vi "Diff_Drive_Sim.vi"() -> ()   [LabVIEW 2019]
uses:
  Sim_Diff_Drive_Globals.vi
panel:
  out "IMU angle(Degrees)":dbl
  out "Left Wheel Position":dbl
  out "Right Wheel Position":dbl
  in  "turning_friction":dbl
  in  "J":dbl
  in  "initial IMU value(degrees)":dbl=0.01
  in  "wheel_base_length":dbl=0.01
  in  "wheel_mass":dbl
  in  "Wheel_friction":dbl
  in  "kinematics delta t (s)":dbl=0.01
  in  "left_wheel_init":dbl
  in  "right_wheel_init":dbl
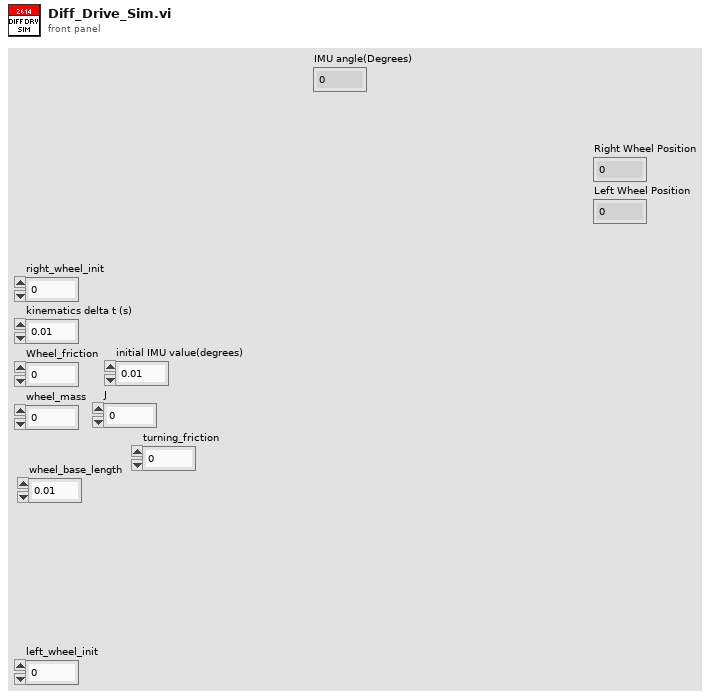
[diagram p1: front panel]
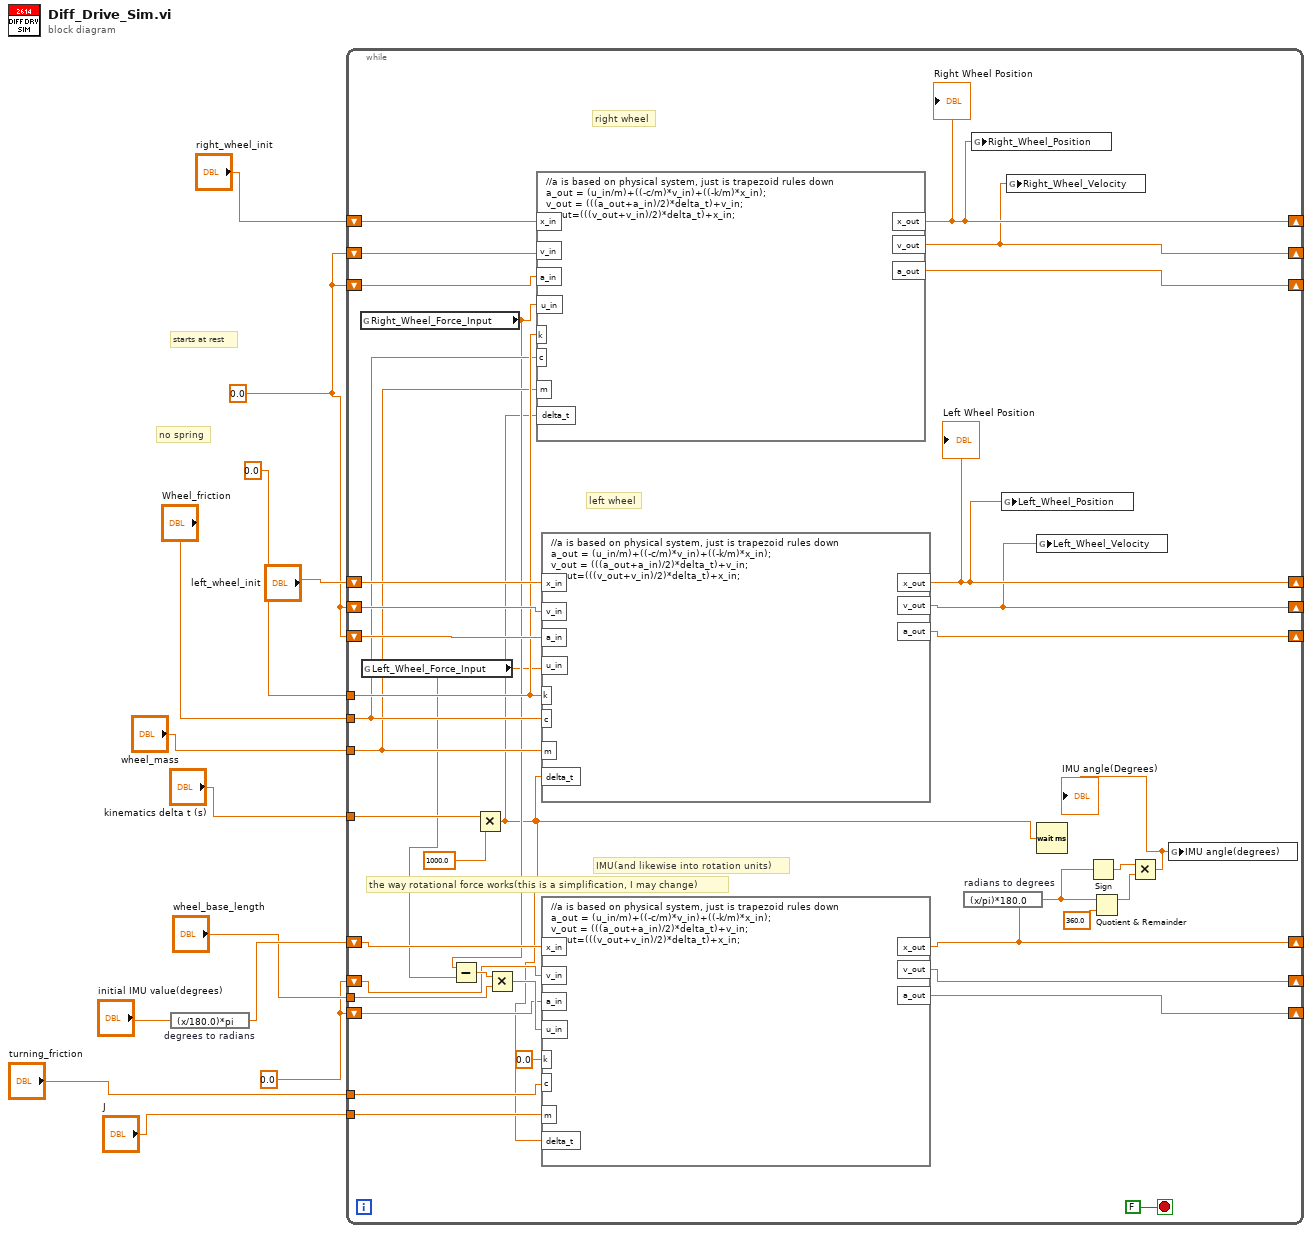
[diagram p0: block diagram]
diagram:
  w3 = 0.0 ("initial IMU value(degrees)")
  w11 = 0.0 ("input variable")
  # "no spring"
  # "starts at rest"
  n1 = expression code="(x/180.0)*pi" "degrees to radians"("initial IMU value(degrees)") -> (w5:dbl)
  n2 = while {
    shift-right: [w37] -> _
    shift-left: w11 -> [w49]
    shift-right: [w35] -> _
    shift-left: w11 -> [w48]
    shift-right: [w44] -> _
    shift-left: w11 -> [w47]
    shift-right: [w45] -> _
    shift-left: w11 -> [w46]
    shift-right: [w38] -> _
    shift-left: "right_wheel_init" -> [w51]
    shift-right: [w36] -> _
    shift-left: "left_wheel_init" -> [w50]
    tunnel: 0.0 ("input variable") -> [w43]
    tunnel: "kinematics delta t (s)" -> [w41]
    tunnel: "Wheel_friction" -> [w40]
    tunnel: "wheel_mass" -> [w39]
    shift-right: [w19] -> _
    shift-left: w5 -> [w34]
    shift-right: [w26] -> _
    shift-left: w3 -> [w28]
    shift-right: [w25] -> _
    shift-left: w3 -> [w27]
    tunnel: "wheel_base_length" -> [w30]
    tunnel: "J" -> [w24]
    tunnel: "turning_friction" -> [w22]
    stop <- FALSE stop-if-true
    # "the way rotational force works(this is a simplification, I may change)"
    # "IMU(and likewise into rotation units)"
    # "left wheel"
    # "right wheel"
    n3 = global read "Sim_Diff_Drive_Globals.vi" "Right_Wheel_Force_Input"() -> (w33:dbl)
    n4 = global read "Sim_Diff_Drive_Globals.vi" "Left_Wheel_Force_Input"() -> (w32:dbl)
    n5 = Subtract(x=w33, y=w32) -> (x-y=w31:dbl)
    n6 = Multiply(x=w41, y=1000.0) -> (x*y=w21:dbl)
    n7 = Multiply(x=w31, y=w30) -> (x*y=w29:dbl)
    n8 = formula code="//a is based on physical system, just is trapezoid rules down\na_out = (u_in/m)+((-c/m)*v_in)+((-k/m)*x_in);\nv_out = (((a_out+a_in)/2)*delta_t)+v_in;\nx_out=(((v_out+v_in)/2)*delta_t)+x_in;"("x_in"=w51, "v_in"=w49, "a_in"=w46, "u_in"=w33, "k"=w43, "c"=w40, "m"=w39, "delta_t"=w21) -> ("x_out"=w38:dbl, "v_out"=w37:dbl, "a_out"=w45:dbl)
    "Right Wheel Position" <- w38
    n9 = formula code="//a is based on physical system, just is trapezoid rules down\na_out = (u_in/m)+((-c/m)*v_in)+((-k/m)*x_in);\nv_out = (((a_out+a_in)/2)*delta_t)+v_in;\nx_out=(((v_out+v_in)/2)*delta_t)+x_in;"("x_in"=w50, "v_in"=w48, "a_in"=w47, "u_in"=w32, "k"=w43, "c"=w40, "m"=w39, "delta_t"=w21) -> ("x_out"=w36:dbl, "v_out"=w35:dbl, "a_out"=w44:dbl)
    "Left Wheel Position" <- w36
    n10 = formula code="//a is based on physical system, just is trapezoid rules down\na_out = (u_in/m)+((-c/m)*v_in)+((-k/m)*x_in);\nv_out = (((a_out+a_in)/2)*delta_t)+v_in;\nx_out=(((v_out+v_in)/2)*delta_t)+x_in;"("x_in"=w34, "v_in"=w28, "a_in"=w27, "u_in"=w29, "k"=0.0 ("input variable"), "c"=w22, "m"=w24, "delta_t"=w21) -> ("x_out"=w19:dbl, "v_out"=w26:dbl, "a_out"=w25:dbl)
    n11 = expression code="(x/pi)*180.0" "radians to degrees"(w19) -> (w17:dbl)
    n12 = global write "Sim_Diff_Drive_Globals.vi" "Right_Wheel_Position"(w38) -> ()
    n13 = global write "Sim_Diff_Drive_Globals.vi" "Left_Wheel_Position"(w36) -> ()
    n14 = global write "Sim_Diff_Drive_Globals.vi" "Right_Wheel_Velocity"(w37) -> ()
    n15 = global write "Sim_Diff_Drive_Globals.vi" "Left_Wheel_Velocity"(w35) -> ()
    n16 = Wait (ms)(milliseconds to wait=w21) -> ()  [unwired: 1 out]
    n17 = Sign(1:w17) -> (0:w16:dbl)
    n18 = Quotient & Remainder(x=w17, y=360.0) -> (x-y*floor(x/y)=w15:dbl)  [unwired: 1 out]
    n19 = Multiply(x=w16, y=w15) -> (x*y=w14:dbl)
    "IMU angle(Degrees)" <- w14
    n20 = global write "Sim_Diff_Drive_Globals.vi" "IMU angle(degrees)"(w14) -> ()
  }
